vi "test_libssh2_userauth_banner.vi"() -> ()   [LabVIEW 2013, in "libssh2_integration_tests.lvlib"]
uses:
  libssh2_integration_tests.lvlib
  libssh2/libssh2_init_default.vi
  libssh2/libssh2_session_handshake_tcp.vi
  libssh2/libssh2.lvlib
  <vilib>/addons/_JKI Toolkits/Caraya/classes/Test/Test.lvclass
  support/support.lvlib
  <vilib>/addons/_JKI Toolkits/Caraya/classes/Assert/Assert.lvclass
panel:
  out "error out":errorcluster
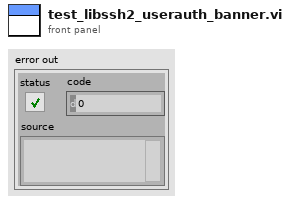
[diagram p1: front panel]
types:
  T1 = typedef "libssh2.lvlib/Session Refnum.ctl" = refnum<k1>
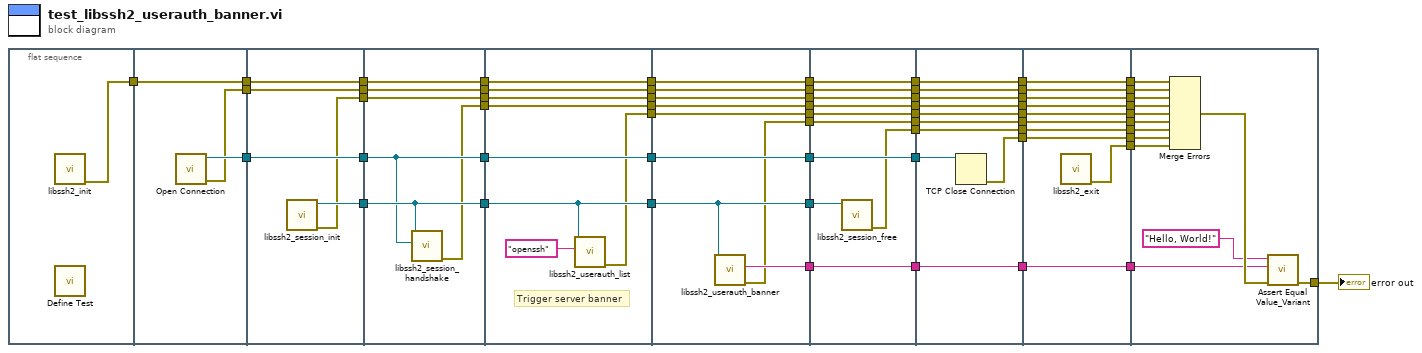
[diagram p0: block diagram]
diagram:
  n1 = flat-sequence {
    tunnel: [w61] -> w60
    tunnel: [w64] -> w59
    tunnel: w60 -> [w63]
    tunnel: [w63] -> w58
    tunnel: [w62] -> w57
    tunnel: w59 -> [w69]
    tunnel: [w69] -> w30
    tunnel: w58 -> [w68]
    tunnel: [w68] -> w29
    tunnel: w57 -> [w67]
    tunnel: [w67] -> w28
    tunnel: [w66] -> w27
    tunnel: [w65] -> w26
    tunnel: w30 -> [w71]
    tunnel: [w71] -> w45
    tunnel: w29 -> [w75]
    tunnel: [w75] -> w44
    tunnel: w28 -> [w74]
    tunnel: [w74] -> w43
    tunnel: [w73] -> w42
    tunnel: w27 -> [w73]
    tunnel: w26 -> [w72]
    tunnel: [w72] -> w41
    tunnel: [w70] -> w40
    tunnel: w45 -> [w83]
    tunnel: [w83] -> w22
    tunnel: w44 -> [w82]
    tunnel: [w82] -> w20
    tunnel: w43 -> [w81]
    tunnel: [w81] -> w18
    tunnel: w42 -> [w78]
    tunnel: w41 -> [w80]
    tunnel: [w80] -> w16
    tunnel: w40 -> [w79]
    tunnel: [w79] -> w14
    tunnel: [w78] -> w12
    tunnel: [w76] -> w9
    tunnel: w22 -> [w92]
    tunnel: [w92] -> w21
    tunnel: w20 -> [w91]
    tunnel: [w91] -> w19
    tunnel: w18 -> [w90]
    tunnel: [w90] -> w17
    tunnel: w16 -> [w89]
    tunnel: [w89] -> w15
    tunnel: w14 -> [w88]
    tunnel: [w88] -> w13
    tunnel: w12 -> [w87]
    tunnel: [w87] -> w11
    tunnel: [w86] -> w10
    tunnel: w9 -> [w85]
    tunnel: [w85] -> w8
    tunnel: [w84] -> w4
    tunnel: w21 -> [w102]
    tunnel: [w102] -> w39
    tunnel: w19 -> [w101]
    tunnel: [w101] -> w38
    tunnel: w17 -> [w100]
    tunnel: [w100] -> w37
    tunnel: w15 -> [w99]
    tunnel: [w99] -> w36
    tunnel: w13 -> [w98]
    tunnel: [w98] -> w35
    tunnel: [w97] -> w32
    tunnel: [w95] -> w23
    tunnel: w11 -> [w96]
    tunnel: w10 -> [w95]
    tunnel: w8 -> [w94]
    tunnel: [w94] -> w7
    tunnel: w4 -> [w93]
    tunnel: [w93] -> w3
    tunnel: w39 -> [w112]
    tunnel: w38 -> [w111]
    tunnel: [w111] -> w56
    tunnel: w37 -> [w110]
    tunnel: [w110] -> w55
    tunnel: [w109] -> w54
    tunnel: w36 -> [w108]
    tunnel: [w108] -> w53
    tunnel: w35 -> [w107]
    tunnel: [w107] -> w52
    tunnel: [w106] -> w33
    tunnel: w32 -> [w106]
    tunnel: [w105] -> w24
    tunnel: w23 -> [w105]
    tunnel: w7 -> [w104]
    tunnel: [w104] -> w6
    tunnel: w3 -> [w103]
    tunnel: [w103] -> w2
    tunnel: w56 -> [w122]
    tunnel: [w122] -> w51
    tunnel: w55 -> [w121]
    tunnel: [w121] -> w50
    tunnel: w54 -> [w120]
    tunnel: [w120] -> w49
    tunnel: [w119] -> w48
    tunnel: w53 -> [w118]
    tunnel: [w118] -> w47
    tunnel: w52 -> [w117]
    tunnel: [w117] -> w46
    tunnel: [w116] -> w34
    tunnel: w33 -> [w116]
    tunnel: [w115] -> w25
    tunnel: w24 -> [w115]
    tunnel: w6 -> [w114]
    tunnel: [w114] -> w5
    tunnel: w2 -> [w113]
    tunnel: [w113] -> w1
    tunnel: w51 -> [w135]
    tunnel: w50 -> [w134]
    tunnel: w49 -> [w133]
    tunnel: w48 -> [w132]
    tunnel: w47 -> [w131]
    tunnel: [w129] -> w31
    tunnel: w46 -> [w128]
    tunnel: w34 -> [w127]
    tunnel: w25 -> [w124]
    tunnel: w5 -> [w126]
    tunnel: w1 -> [w125]
    frame #0 {
      n2 = call-poly "libssh2_init.vi"() -> ("error out"=w61:errorcluster)  [unwired: 11 in]
      n3 = call <vilib>:"Define Test.vi"() -> ()  [unwired: 10 in, 2 out]
    }
    frame #1 {
      n4 = call "Open Connection.vi"() -> ("error out"=w62:errorcluster, "connection ID"=w64:refnum<k5>)  [unwired: 10 in]
    }
    frame #2 {
      n5 = call "libssh2_session_init.vi"() -> ("error out"=w65:errorcluster, "session"=w66:T1)  [unwired: 10 in]
    }
    frame #3 {
      n6 = call-poly "libssh2_session_handshake.vi"("tcp connection"=w71, "session"=w73) -> ("error out"=w70:errorcluster)  [unwired: 9 in]
    }
    frame #4 {
      # "Trigger server banner"
      n7 = call "libssh2_userauth_list.vi"("username"="openssh", "session"=w78) -> ("error out"=w76:errorcluster)  [unwired: 8 in, 1 out]
    }
    frame #5 {
      n8 = call "libssh2_userauth_banner.vi"("session"=w87) -> ("error out"=w84:errorcluster, "banner"=w86:string)  [unwired: 9 in]
    }
    frame #6 {
      n9 = call "libssh2_session_free.vi"("session"=w96) -> ("error out"=w97:errorcluster)  [unwired: 10 in]
    }
    frame #7 {
      n10 = TCP Close Connection(connection ID=w112) -> (error out=w109:errorcluster)  [unwired: 2 in, 1 out]
    }
    frame #8 {
      n11 = call "libssh2_exit.vi"() -> ("error out"=w119:errorcluster)  [unwired: 11 in]
    }
    frame #9 {
      n12 = Merge Errors(w135, w134, w131, w128, w126, w125, w127, w133, w132) -> (w130:errorcluster)
      n13 = call <vilib>:"Assert Equal Value_Variant.vi"("error in (no error)"=w130, "Y"=w124, "X"="Hello, World!" ("banner")) -> ("error out"=w129:errorcluster)  [unwired: 7 in, 1 out]
    }
  }
  "error out" <- w31
